vi "Open Sensors and Actuators.vi"   [LabVIEW 2014]
uses:
  <vilib>/Rock Robotics/SystemInterfaces/DIO/FPGA_DIOPWMChannel.ctl
  <vilib>/Rock Robotics/SystemInterfaces/AI/FPGA_AIChannel.ctl
  <vilib>/Rock Robotics/WPI/Joystick/WPI_JoystickDeviceEnum.ctl
  <vilib>/Rock Robotics/SystemInterfaces/DIO/FPGA_DIOChannel.ctl
  <vilib>/Rock Robotics/WPI/Solenoid/WPI_SolenoidChannel.ctl
  <vilib>/Rock Robotics/SystemInterfaces/Typedef/FPGA_TypedefAnalogModule.ctl
  <vilib>/Rock Robotics/WPI/MotorControl/WPI_MotorControlOpen Talon.vi
  <vilib>/Rock Robotics/WPI/Counter/WPI_CounterDigitalInputToDigitalSource.vi
  <vilib>/Rock Robotics/WPI/Solenoid/WPI_SolenoidOpenSingle.vi
  <vilib>/Rock Robotics/WPI/Counter/WPI_CounterOpen UpDown Mode.vi
  <vilib>/Rock Robotics/WPI/Switch/WPI_SwitchOpenLimit.vi
  Global RefNums.vi
  <vilib>/Rock Robotics/WPI/Compressor/WPI_CompressorGetSetRefNum.vi
  _Dependencies/NavX/navX-MXP IMU.lvlib
types:
  T1 = typedef "FPGA_AIChannel.ctl" = enum8{"AI 0", "AI 1", "AI 2", "AI 3", "AI MXP 0", "AI MXP 1", "AI MXP 2", "AI MXP 3", "Invalid"}
  T2 = typedef "FPGA_TypedefAnalogModule.ctl" = enum16{"Controller 1"}
  T3 = typedef "FPGA_DIOPWMChannel.ctl" = enum8{"PWM 0", "PWM 1", "PWM 2", "PWM 3", "PWM 4", "PWM 5", "PWM 6", "PWM 7", "PWM 8", "PWM 9", "PWM MXP 0", "PWM MXP 1", "PWM MXP 2", "PWM MXP 3", "PWM MXP 4", "PWM MXP 5", "PWM MXP 6", "PWM MXP 7", "PWM MXP 8", "PWM MXP 9", "Invalid"}
  T4 = typedef "FPGA_DIOChannel.ctl" = enum8{"DIO 0", "DIO 1", "DIO 2", "DIO 3", "DIO 4", "DIO 5", "DIO 6", "DIO 7", "DIO 8", "DIO 9", "DIO MXP 0", "DIO MXP 1", "DIO MXP 2", "DIO MXP 3", "DIO MXP 4", "DIO MXP 5", "DIO MXP 6", "DIO MXP 7", "DIO MXP 8", "DIO MXP 9", "DIO MXP 10", "DIO MXP 11", "DIO MXP 12", "DIO MXP 13", "DIO MXP 14", "DIO MXP 15", "Invalid"}
  T5 = enum16{"Rising Edge", "Falling Edge", "Raising & Falling Edge", "Disabled"}
  T6 = typedef "WPI_SolenoidChannel.ctl" = enum8{"Solenoid 0", "Solenoid 1", "Solenoid 2", "Solenoid 3", "Solenoid 4", "Solenoid 5", "Solenoid 6", "Solenoid 7", "Invalid"}
  T7 = typedef "WPI_JoystickDeviceEnum.ctl" = enum16{"USB 0", "USB 1", "USB 2", "USB 3", "USB 4", "USB 5"}
  T8 = typedef "WPI_MotorControlDeviceRef.ctl" = cluster{"DeviceStatus":errorcluster, "Type":T9, "PWM":cluster{"Controller":T10, "PWM Channel":T3, "DeadBand":T11}, "CAN":cluster{"Device Number":u8, "Control Mode":T12, "Semaphore":T13, "Max Vout":dbl, "TalonSRX Control Mode":T14}, "Invert":bool, "TransformRef":T15, "InvTransformRef":T15}
  T9 = typedef "WPI_MotorControlType.ctl" = enum16{"PWM", "CAN", "CANTalonSRX"}
  T10 = typedef "FPGA_TypedefDigitalModule.ctl" = enum16{"Controller 1"}
  T11 = typedef "WPI_PWMDeadband.ctl" = cluster{"Name":string, "maxPositivePwm":i32, "minPositivePwm":i32, "centerPwm":i32, "maxNegativePwm":i32, "minNegativePwm":i32, "angularRange":u16}
  T12 = typedef "WPI_CANJaguar_ControlMode.ctl" = enum8{"Percent VBus", "Current", "Speed", "Position", "Voltage"}
  T13 = typedef "Semaphore RefNum" = refnum<k1>
  T14 = typedef "WPI_CANTalonSRX_APIControlMode.ctl" = enum8{"Percent VBus", "Speed", "Position", "Slave", "Unchanged / Invalid"}
  T15 = typedef "WPI_PWMTransform_ConPane.ctl" = refnum<vi>
  T16 = typedef "WPI_DigitalInputDevRef.ctl" = cluster{"DevStatus":errorcluster, "DIO Channel":T4, "Controller":T10}
  T17 = typedef "FPGA_CounterEncoderSourceConvertionLVSourceType.ctl" = cluster{"DevStatus":errorcluster, "AnalogTriggerMode?":bool, "DigitalMode":cluster{"Controller":T10, "DIO Channel":T18}, "AnalogTriggerMode":cluster{"AnalogTriggerIndex":T19, "OutputType":T20}}
  T18 = typedef "FPGA_DIODigitalSourceChannel.ctl" = enum8{"DIO 0", "DIO 1", "DIO 2", "DIO 3", "DIO 4", "DIO 5", "DIO 6", "DIO 7", "DIO 8", "DIO 9", "DIO MXP 0", "DIO MXP 1", "DIO MXP 2", "DIO MXP 3", "DIO MXP 4", "DIO MXP 5", "DIO MXP 6", "DIO MXP 7", "DIO MXP 8", "DIO MXP 9", "DIO MXP 10", "DIO MXP 11", "DIO MXP 12", "DIO MXP 13", "DIO MXP 14", "DIO MXP 15", "Disabled"}
  T19 = typedef "FPGA_AnalogTriggerIndex.ctl" = enum8{"Trig 0", "Trig 1", "Trig 2", "Trig 3", "Trig 4", "Trig 5", "Trig 6", "Trig 7", "Invalid"}
  T20 = typedef "FPGA_AnalogTriggerOutType.ctl" = enum16{"InWindow", "TriggerState", "Rising", "Falling"}
  T21 = typedef "WPI_EncoderDevRef.ctl" = cluster{"DevStatus":errorcluster, "EncoderIndex":T22, "CounterIndex":T23, "DistancePerCount":dbl, "Decoding Type":T24}
  T22 = typedef "FPGA_EncoderIdx.ctl" = enum8{"Enc 0", "Enc 1", "Enc 2", "Enc 3", "Enc 4", "Enc 5", "Enc 6", "Enc 7", "Invalid"}
  T23 = typedef "FPGA_CounterCtrSystemIndex.ctl" = enum8{"Ctr 0", "Ctr 1", "Ctr 2", "Ctr 3", "Ctr 4", "Ctr 5", "Ctr 6", "Ctr 7", "Invalid"}
  T24 = typedef "WPI_EncoderType.ctl" = enum16{"1x", "2x", "4x"}
  T25 = typedef "navX-MXP IMU.lvlib/navX Device TypeDef.ctl" = cluster{"navX Interface Protocol":T26, "navX Interface Protocol TypeDefs":cluster{"SPIDevRef":T27, "I2CDevRef":T29}, "navX System Information":cluster{"Board Information":T31, "Status":T32, "Offsets":T36}, "navX Common Information":cluster{"Update Rate (4Hz-60Hz)":T37, "refnum name":string, "error":errorcluster}}
  T26 = typedef "navX-MXP IMU.lvlib/navX Interface Protocol.ctl" = enum16{"SPI", "I2C"}
  T27 = typedef "WPI_SPIDevRef.ctl" = cluster{"DevStatus":errorcluster, "Handle":i32, "Controller":T10, "SPI Bus":T28}
  T28 = typedef "spi_bus.ctl" = enum16{"SPI On-Board, CS0", "SPI On-Board, CS1", "SPI On-Board, CS2", "SPI On-Board, CS3", "SPI MXP", "Invalid"}
  T29 = typedef "WPI_I2CDevRef.ctl" = cluster{"DevStatus":errorcluster, "Controller":T10, "Device Address":u8, "Handle":i32, "I2C Bus":T30}
  T30 = typedef "i2c_bus.ctl" = enum16{"I2C On-Board", "I2C MXP", "Invalid"}
  T31 = typedef "navX-MXP IMU.lvlib/navX Board Information.ctl" = cluster{"WhoAmI (50 | 0x32)":u8, "Board Revision":u8, "Firmware Major Version":u8, "Firmware Minor Version":u8}
  T32 = typedef "navX-MXP IMU.lvlib/navX Status Data.ctl" = cluster{"Update Rate Hz":u8, "Accelerometer Full-Scale Range":u8, "Gyro Full-Scale Range":u16, "NAVX_OP_STATUS":T33, "NAVX_CAL_STATUS":T34, "NAVX_SELFTEST_STATUS":u8, "NAVX_SENSOR_STATUS":T35}
  T33 = typedef "navX-MXP IMU.lvlib/navX NAVX_OP_STATUS.ctl" = u8
  T34 = typedef "navX-MXP IMU.lvlib/navX NAVX_CAL_STATUS.ctl" = u8
  T35 = typedef "navX-MXP IMU.lvlib/navX NAVX_SENSOR_STATUS.ctl" = cluster{"MOVING":bool, "YAW_STABLE":bool, "MAG_DISTURBANCE":bool, "ALTITUDE_VALID":bool, "SEALEVEL_PRESS_SET":bool, "FUSED_HEADING_VALID":bool}
  T36 = typedef "navX-MXP IMU.lvlib/navX Offsets Data.ctl" = cluster{"Yaw":dbl, "Quat W":dbl, "Quat X":dbl, "Quat Y":dbl, "Quat Z":dbl}
  T37 = typedef "navX-MXP IMU.lvlib/navX Update Rate.ctl" = u8
  T38 = typedef "WPI_JoystickDevRef.ctl" = cluster{"Device":T7}
  T39 = typedef "WPI_AnalogChannelDevRef.ctl" = cluster{"DevStatus":errorcluster, "Controller":T2, "Analog Channel":T1}
  T40 = typedef "WPI_SolenoidDevRef.ctl" = cluster{"DevStatus":errorcluster, "Pneumatics Control Module":u8, "Forward Solenoid Channel":T6, "Reverse Solenoid Channel":T6}
  T41 = typedef "WPI_CounterDevRef.ctl" = cluster{"DevStatus":errorcluster, "CntIndex":T23}
  T42 = typedef "WPI_CompressorDevRef.ctl" = cluster{"DevStatus":errorcluster, "Pneumatics Control Module":u8}
  T43 = typedef "WPI_SwitchDevRef.ctl" = cluster{"DevStatus":errorcluster, "DIO Channel":T4, "Controller":T10, "CntIndex":T23, "Normally Closed":bool}
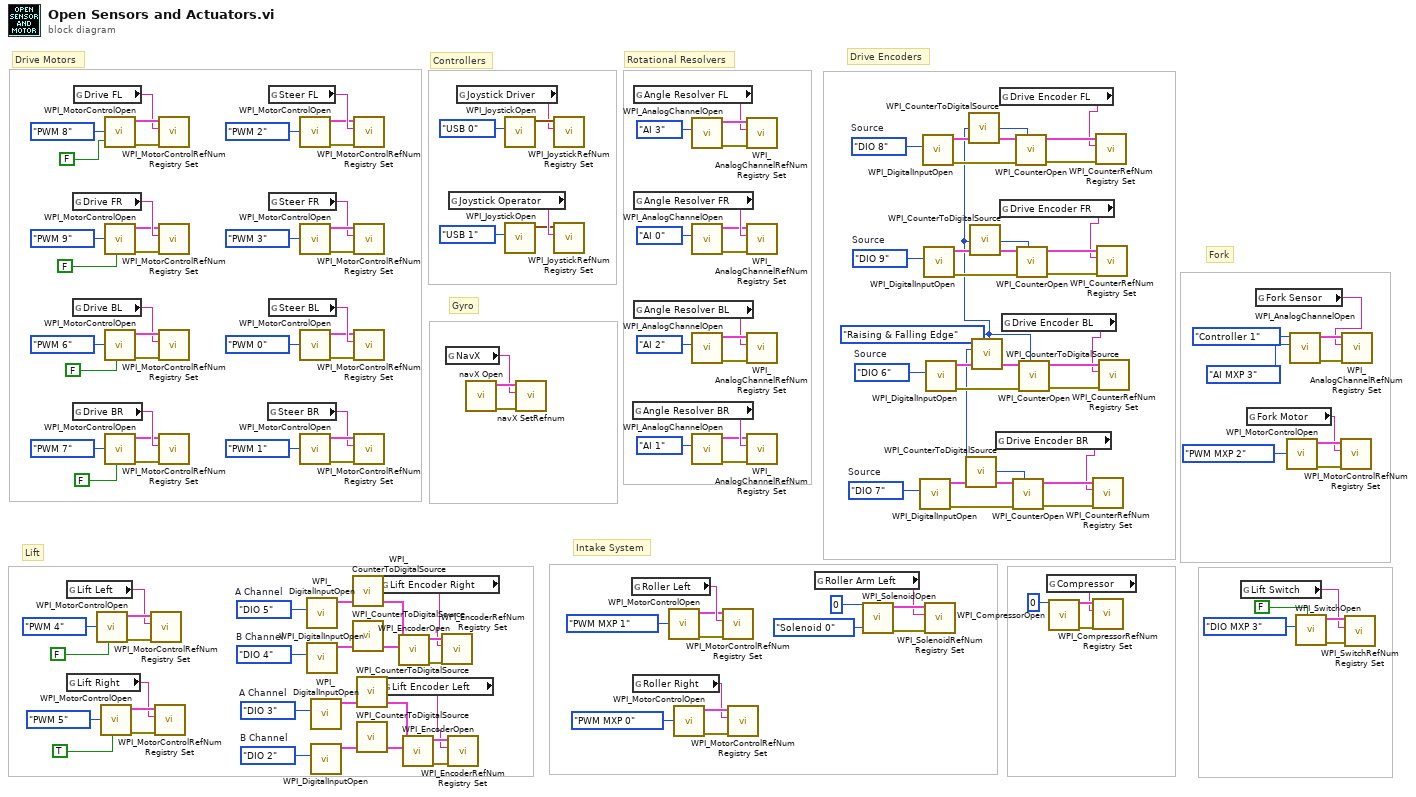
[diagram p0: block diagram]
diagram:
  w15 = T5."Raising & Falling Edge" ("UpEdge")
  w25 = FPGA_DIOChannel."DIO 7"  # Source
  w32 = FPGA_DIOChannel."DIO 6"  # Source
  w39 = FPGA_DIOChannel."DIO 9"  # Source
  w67 = FPGA_DIOChannel."DIO 2"  # B Channel
  w66 = FPGA_DIOChannel."DIO 3"  # A Channel
  w73 = FPGA_DIOChannel."DIO 4"  # B Channel
  w72 = FPGA_DIOChannel."DIO 5"  # A Channel
  w94 = FPGA_DIOChannel."DIO 8"  # Source
  # "Fork"
  # "Intake System"
  # "Gyro"
  # "Drive Encoders"
  # "Lift"
  # "Drive Motors"
  # "Controllers"
  # "Rotational Resolvers"
  n1 = global read "Global RefNums.vi" "Lift Left"() -> (w83:string)
  n2 = global read "Global RefNums.vi" "Lift Right"() -> (w79:string)
  n3 = global read "Global RefNums.vi" "Drive FR"() -> (w141:string)
  n4 = global read "Global RefNums.vi" "Drive BL"() -> (w136:string)
  n5 = global read "Global RefNums.vi" "Drive BR"() -> (w133:string)
  n6 = global read "Global RefNums.vi" "Drive FL"() -> (w144:string)
  n7 = call-poly <vilib>:"WPI_MotorControlOpen.vi"("Invert"=FALSE, "PWM Channel"=FPGA_DIOPWMChannel."PWM 4") -> ("error out"=w84:errorcluster, "MotorControlDeviceRef"=w85:T8)  [unwired: 8 in]
  n8 = call-poly <vilib>:"WPI_MotorControlOpen.vi"("Invert"=TRUE, "PWM Channel"=FPGA_DIOPWMChannel."PWM 5") -> ("error out"=w80:errorcluster, "MotorControlDeviceRef"=w81:T8)  [unwired: 8 in]
  n9 = call-poly <vilib>:"WPI_MotorControlOpen.vi"("Invert"=FALSE, "PWM Channel"=FPGA_DIOPWMChannel."PWM 8") -> ("error out"=w145:errorcluster, "MotorControlDeviceRef"=w146:T8)  [unwired: 8 in]
  n10 = call-poly <vilib>:"WPI_MotorControlOpen.vi"("Invert"=FALSE, "PWM Channel"=FPGA_DIOPWMChannel."PWM 9") -> ("error out"=w140:errorcluster, "MotorControlDeviceRef"=w139:T8)  [unwired: 8 in]
  n11 = call-poly <vilib>:"WPI_MotorControlOpen.vi"("Invert"=FALSE, "PWM Channel"=FPGA_DIOPWMChannel."PWM 6") -> ("error out"=w137:errorcluster, "MotorControlDeviceRef"=w138:T8)  [unwired: 8 in]
  n12 = call-poly <vilib>:"WPI_MotorControlOpen.vi"("Invert"=FALSE, "PWM Channel"=FPGA_DIOPWMChannel."PWM 7") -> ("error out"=w132:errorcluster, "MotorControlDeviceRef"=w131:T8)  [unwired: 8 in]
  n13 = call <vilib>:"WPI_MotorControlRefNum Registry Set.vi"("error in (no error)"=w84, "refnum name"=w83, "MotorControlDevRef"=w85) -> ()  [unwired: 7 in, 2 out]
  n14 = call <vilib>:"WPI_MotorControlRefNum Registry Set.vi"("error in (no error)"=w80, "refnum name"=w79, "MotorControlDevRef"=w81) -> ()  [unwired: 7 in, 2 out]
  n15 = call <vilib>:"WPI_MotorControlRefNum Registry Set.vi"("error in (no error)"=w145, "refnum name"=w144, "MotorControlDevRef"=w146) -> ()  [unwired: 7 in, 2 out]
  n16 = call <vilib>:"WPI_MotorControlRefNum Registry Set.vi"("error in (no error)"=w140, "refnum name"=w141, "MotorControlDevRef"=w139) -> ()  [unwired: 7 in, 2 out]
  n17 = call <vilib>:"WPI_MotorControlRefNum Registry Set.vi"("error in (no error)"=w137, "refnum name"=w136, "MotorControlDevRef"=w138) -> ()  [unwired: 7 in, 2 out]
  n18 = call <vilib>:"WPI_MotorControlRefNum Registry Set.vi"("error in (no error)"=w132, "refnum name"=w133, "MotorControlDevRef"=w131) -> ()  [unwired: 7 in, 2 out]
  n19 = global read "Global RefNums.vi" "Steer BR"() -> (w128:string)
  n20 = global read "Global RefNums.vi" "Steer FL"() -> (w117:string)
  n21 = global read "Global RefNums.vi" "Steer FR"() -> (w120:string)
  n22 = global read "Global RefNums.vi" "Steer BL"() -> (w125:string)
  n23 = call-poly <vilib>:"WPI_MotorControlOpen.vi"("PWM Channel"=FPGA_DIOPWMChannel."PWM 2") -> ("error out"=w116:errorcluster, "MotorControlDeviceRef"=w115:T8)  [unwired: 9 in]
  n24 = call-poly <vilib>:"WPI_MotorControlOpen.vi"("PWM Channel"=FPGA_DIOPWMChannel."PWM 3") -> ("error out"=w121:errorcluster, "MotorControlDeviceRef"=w122:T8)  [unwired: 9 in]
  n25 = call-poly <vilib>:"WPI_MotorControlOpen.vi"("PWM Channel"=FPGA_DIOPWMChannel."PWM 0") -> ("error out"=w124:errorcluster, "MotorControlDeviceRef"=w123:T8)  [unwired: 9 in]
  n26 = call-poly <vilib>:"WPI_MotorControlOpen.vi"("PWM Channel"=FPGA_DIOPWMChannel."PWM 1") -> ("error out"=w129:errorcluster, "MotorControlDeviceRef"=w130:T8)  [unwired: 9 in]
  n27 = call <vilib>:"WPI_DigitalInputOpen.vi"("DIO Channel"=w72) -> ("DigitalInputDevRef"=w69:T16)  [unwired: 2 in, 8 out]
  n28 = call <vilib>:"WPI_DigitalInputOpen.vi"("DIO Channel"=w73) -> ("DigitalInputDevRef"=w70:T16)  [unwired: 2 in, 8 out]
  n29 = call <vilib>:"WPI_DigitalInputOpen.vi"("DIO Channel"=w66) -> ("DigitalInputDevRef"=w63:T16)  [unwired: 2 in, 8 out]
  n30 = call <vilib>:"WPI_DigitalInputOpen.vi"("DIO Channel"=w67) -> ("DigitalInputDevRef"=w64:T16)  [unwired: 2 in, 8 out]
  n31 = call-poly <vilib>:"WPI_CounterToDigitalSource.vi"("DigitalInputDevRef"=w69) -> ("Digital Source"=w68:T17)  [unwired: 6 out]
  n32 = call-poly <vilib>:"WPI_CounterToDigitalSource.vi"("DigitalInputDevRef"=w70) -> ("Digital Source"=w71:T17)  [unwired: 6 out]
  n33 = call <vilib>:"WPI_MotorControlRefNum Registry Set.vi"("error in (no error)"=w116, "refnum name"=w117, "MotorControlDevRef"=w115) -> ()  [unwired: 7 in, 2 out]
  n34 = call <vilib>:"WPI_MotorControlRefNum Registry Set.vi"("error in (no error)"=w121, "refnum name"=w120, "MotorControlDevRef"=w122) -> ()  [unwired: 7 in, 2 out]
  n35 = call <vilib>:"WPI_MotorControlRefNum Registry Set.vi"("error in (no error)"=w124, "refnum name"=w125, "MotorControlDevRef"=w123) -> ()  [unwired: 7 in, 2 out]
  n36 = call <vilib>:"WPI_MotorControlRefNum Registry Set.vi"("error in (no error)"=w129, "refnum name"=w128, "MotorControlDevRef"=w130) -> ()  [unwired: 7 in, 2 out]
  n37 = call-poly <vilib>:"WPI_CounterToDigitalSource.vi"("DigitalInputDevRef"=w63) -> ("Digital Source"=w62:T17)  [unwired: 6 out]
  n38 = call-poly <vilib>:"WPI_CounterToDigitalSource.vi"("DigitalInputDevRef"=w64) -> ("Digital Source"=w65:T17)  [unwired: 6 out]
  n39 = global read "Global RefNums.vi" "Lift Encoder Right"() -> (w56:string)
  n40 = global read "Global RefNums.vi" "Lift Encoder Left"() -> (w57:string)
  n41 = call <vilib>:"WPI_EncoderOpen.vi"("BSource"=w71, "ASource"=w68) -> ("error out"=w61:errorcluster, "EncoderDevRef"=w60:T21)  [unwired: 6 in, 2 out]
  n42 = call <vilib>:"WPI_EncoderOpen.vi"("BSource"=w65, "ASource"=w62) -> ("error out"=w59:errorcluster, "EncoderDevRef"=w58:T21)  [unwired: 6 in, 2 out]
  n43 = call <vilib>:"WPI_EncoderRefNum Registry Set.vi"("error in (no error)"=w61, "refnum name"=w56, "EncoderDevRef"=w60) -> ()  [unwired: 7 in, 2 out]
  n44 = global read "Global RefNums.vi" "NavX"() -> (w86:string)
  n45 = call <vilib>:"WPI_EncoderRefNum Registry Set.vi"("error in (no error)"=w59, "refnum name"=w57, "EncoderDevRef"=w58) -> ()  [unwired: 7 in, 2 out]
  n46 = global read "Global RefNums.vi" "Joystick Operator"() -> (w113:string)
  n47 = global read "Global RefNums.vi" "Joystick Driver"() -> (w114:string)
  n48 = call "navX Open.vi"() -> ("error out"=w88:errorcluster, "navX Device TypeDef"=w87:T25)  [unwired: 9 in, 1 out]
  n49 = call <vilib>:"WPI_JoystickOpen.vi"("JoystickDevice"=WPI_JoystickDeviceEnum."USB 0") -> ("JoystickDevRef"=w147:T38)  [unwired: 10 in]
  n50 = call <vilib>:"WPI_JoystickOpen.vi"("JoystickDevice"=WPI_JoystickDeviceEnum."USB 1") -> ("JoystickDevRef"=w112:T38)  [unwired: 10 in]
  n51 = call "navX SetRefnum.vi"("error in (no error)"=w88, "refnum name"=w86, "navX Device TypeDef"=w87) -> ()  [unwired: 7 in, 2 out]
  n52 = call <vilib>:"WPI_JoystickRefNum Registry Set.vi"("refnum name"=w114, "JoystickDevRef"=w147) -> ()  [unwired: 8 in, 2 out]
  n53 = call <vilib>:"WPI_JoystickRefNum Registry Set.vi"("refnum name"=w113, "JoystickDevRef"=w112) -> ()  [unwired: 8 in, 2 out]
  n54 = global read "Global RefNums.vi" "Roller Left"() -> (w52:string)
  n55 = global read "Global RefNums.vi" "Angle Resolver BR"() -> (w100:string)
  n56 = global read "Global RefNums.vi" "Roller Right"() -> (w47:string)
  n57 = global read "Global RefNums.vi" "Angle Resolver FL"() -> (w111:string)
  n58 = global read "Global RefNums.vi" "Angle Resolver FR"() -> (w108:string)
  n59 = global read "Global RefNums.vi" "Angle Resolver BL"() -> (w103:string)
  n60 = call-poly <vilib>:"WPI_MotorControlOpen.vi"("PWM Channel"=FPGA_DIOPWMChannel."PWM MXP 1") -> ("error out"=w51:errorcluster, "MotorControlDeviceRef"=w50:T8)  [unwired: 9 in]
  n61 = call-poly <vilib>:"WPI_MotorControlOpen.vi"("PWM Channel"=FPGA_DIOPWMChannel."PWM MXP 0") -> ("error out"=w48:errorcluster, "MotorControlDeviceRef"=w49:T8)  [unwired: 9 in]
  n62 = call <vilib>:"WPI_AnalogChannelOpen.vi"("Analog Channel"=FPGA_AIChannel."AI 3") -> ("error out"=w149:errorcluster, "AIDeviceRef"=w148:T39)  [unwired: 9 in]
  n63 = call <vilib>:"WPI_AnalogChannelOpen.vi"("Analog Channel"=FPGA_AIChannel."AI 0") -> ("error out"=w106:errorcluster, "AIDeviceRef"=w107:T39)  [unwired: 9 in]
  n64 = call <vilib>:"WPI_AnalogChannelOpen.vi"("Analog Channel"=FPGA_AIChannel."AI 2") -> ("error out"=w105:errorcluster, "AIDeviceRef"=w104:T39)  [unwired: 9 in]
  n65 = call <vilib>:"WPI_AnalogChannelOpen.vi"("Analog Channel"=FPGA_AIChannel."AI 1") -> ("error out"=w98:errorcluster, "AIDeviceRef"=w99:T39)  [unwired: 9 in]
  n66 = call <vilib>:"WPI_MotorControlRefNum Registry Set.vi"("error in (no error)"=w51, "refnum name"=w52, "MotorControlDevRef"=w50) -> ()  [unwired: 7 in, 2 out]
  n67 = call <vilib>:"WPI_MotorControlRefNum Registry Set.vi"("error in (no error)"=w48, "refnum name"=w47, "MotorControlDevRef"=w49) -> ()  [unwired: 7 in, 2 out]
  n68 = call <vilib>:"WPI_AnalogChannelRefNum Registry Set.vi"("error in (no error)"=w149, "refnum name"=w111, "AIDeviceRef"=w148) -> ()  [unwired: 7 in, 2 out]
  n69 = call <vilib>:"WPI_AnalogChannelRefNum Registry Set.vi"("error in (no error)"=w106, "refnum name"=w108, "AIDeviceRef"=w107) -> ()  [unwired: 7 in, 2 out]
  n70 = call <vilib>:"WPI_AnalogChannelRefNum Registry Set.vi"("error in (no error)"=w105, "refnum name"=w103, "AIDeviceRef"=w104) -> ()  [unwired: 7 in, 2 out]
  n71 = call <vilib>:"WPI_AnalogChannelRefNum Registry Set.vi"("error in (no error)"=w98, "refnum name"=w100, "AIDeviceRef"=w99) -> ()  [unwired: 7 in, 2 out]
  n72 = global read "Global RefNums.vi" "Roller Arm Left"() -> (w41:string)
  n73 = call-poly <vilib>:"WPI_SolenoidOpen.vi"("Solenoid Channel"=WPI_SolenoidChannel."Solenoid 0", "Pneumatics Control Module (0)"=u8 0) -> ("error out"=w44:errorcluster, "SolenoidDevRef"=w45:T40)  [unwired: 8 in]
  n74 = call <vilib>:"WPI_DigitalInputOpen.vi"("DIO Channel"=w25) -> ("error out"=w21:errorcluster, "DigitalInputDevRef"=w24:T16)  [unwired: 2 in, 7 out]
  n75 = call <vilib>:"WPI_DigitalInputOpen.vi"("DIO Channel"=w94) -> ("error out"=w90:errorcluster, "DigitalInputDevRef"=w93:T16)  [unwired: 2 in, 7 out]
  n76 = call <vilib>:"WPI_DigitalInputOpen.vi"("DIO Channel"=w39) -> ("error out"=w35:errorcluster, "DigitalInputDevRef"=w38:T16)  [unwired: 2 in, 7 out]
  n77 = call <vilib>:"WPI_SolenoidRefNum Registry Set.vi"("error in (no error)"=w44, "refnum name"=w41, "SolenoidDevRef"=w45) -> ()  [unwired: 7 in, 2 out]
  n78 = call <vilib>:"WPI_DigitalInputOpen.vi"("DIO Channel"=w32) -> ("error out"=w28:errorcluster, "DigitalInputDevRef"=w31:T16)  [unwired: 2 in, 7 out]
  n79 = call-poly <vilib>:"WPI_CounterToDigitalSource.vi"("DigitalInputDevRef"=w24) -> ("Digital Source"=w26:T17)  [unwired: 6 out]
  n80 = call-poly <vilib>:"WPI_CounterToDigitalSource.vi"("DigitalInputDevRef"=w93) -> ("Digital Source"=w95:T17)  [unwired: 6 out]
  n81 = call-poly <vilib>:"WPI_CounterToDigitalSource.vi"("DigitalInputDevRef"=w38) -> ("Digital Source"=w40:T17)  [unwired: 6 out]
  n82 = call-poly <vilib>:"WPI_CounterToDigitalSource.vi"("DigitalInputDevRef"=w31) -> ("Digital Source"=w33:T17)  [unwired: 6 out]
  n83 = global read "Global RefNums.vi" "Drive Encoder BR"() -> (w20:string)
  n84 = global read "Global RefNums.vi" "Drive Encoder FL"() -> (w89:string)
  n85 = global read "Global RefNums.vi" "Drive Encoder FR"() -> (w34:string)
  n86 = global read "Global RefNums.vi" "Drive Encoder BL"() -> (w27:string)
  n87 = call-poly <vilib>:"WPI_CounterOpen.vi"("UpEdge"=w15, "error in (no error)"=w21, "Up Source"=w26) -> ("error out"=w22:errorcluster, "CounterDevRef"=w23:T41)  [unwired: 4 in, 3 out]
  n88 = call-poly <vilib>:"WPI_CounterOpen.vi"("UpEdge"=w15, "error in (no error)"=w90, "Up Source"=w95) -> ("error out"=w91:errorcluster, "CounterDevRef"=w92:T41)  [unwired: 4 in, 3 out]
  n89 = call-poly <vilib>:"WPI_CounterOpen.vi"("UpEdge"=w15, "error in (no error)"=w35, "Up Source"=w40) -> ("error out"=w36:errorcluster, "CounterDevRef"=w37:T41)  [unwired: 4 in, 3 out]
  n90 = call-poly <vilib>:"WPI_CounterOpen.vi"("UpEdge"=w15, "error in (no error)"=w28, "Up Source"=w33) -> ("error out"=w29:errorcluster, "CounterDevRef"=w30:T41)  [unwired: 4 in, 3 out]
  n91 = global read "Global RefNums.vi" "Compressor"() -> (w16:string)
  n92 = call <vilib>:"WPI_CompressorOpen.vi"("Pneumatics Control Module (0)"=u8 0) -> ("CompressorDevRef"=w19:T42, "error out"=w18:errorcluster)  [unwired: 13 in]
  n93 = call <vilib>:"WPI_CounterRefNum Registry Set.vi"("error in (no error)"=w22, "refnum name"=w20, "CounterDevRef"=w23) -> ()  [unwired: 7 in, 2 out]
  n94 = call <vilib>:"WPI_CompressorRefNum Registry Set.vi"("error in (no error)"=w18, "refnum name"=w16, "CompressorDevRef"=w19) -> ()  [unwired: 7 in, 2 out]
  n95 = call <vilib>:"WPI_CounterRefNum Registry Set.vi"("error in (no error)"=w91, "refnum name"=w89, "CounterDevRef"=w92) -> ()  [unwired: 7 in, 2 out]
  n96 = call <vilib>:"WPI_CounterRefNum Registry Set.vi"("error in (no error)"=w36, "refnum name"=w34, "CounterDevRef"=w37) -> ()  [unwired: 7 in, 2 out]
  n97 = call <vilib>:"WPI_CounterRefNum Registry Set.vi"("error in (no error)"=w29, "refnum name"=w27, "CounterDevRef"=w30) -> ()  [unwired: 7 in, 2 out]
  n98 = global read "Global RefNums.vi" "Lift Switch"() -> (w11:string)
  n99 = global read "Global RefNums.vi" "Fork Motor"() -> (w7:string)
  n100 = global read "Global RefNums.vi" "Fork Sensor"() -> (w1:string)
  n101 = call-poly <vilib>:"WPI_MotorControlOpen.vi"("PWM Channel"=FPGA_DIOPWMChannel."PWM MXP 2") -> ("error out"=w8:errorcluster, "MotorControlDeviceRef"=w9:T8)  [unwired: 9 in]
  n102 = call <vilib>:"WPI_AnalogChannelOpen.vi"("Analog Channel"=FPGA_AIChannel."AI MXP 3", "Controller"=FPGA_TypedefAnalogModule."Controller 1") -> ("error out"=w4:errorcluster, "AIDeviceRef"=w5:T39)  [unwired: 8 in]
  n103 = call-poly <vilib>:"WPI_SwitchOpen.vi"("Normally Closed"=FALSE, "DIO Channel"=FPGA_DIOChannel."DIO MXP 3") -> ("error out"=w14:errorcluster, "SwitchDevRef"=w13:T43)  [unwired: 8 in]
  n104 = call <vilib>:"WPI_MotorControlRefNum Registry Set.vi"("error in (no error)"=w8, "refnum name"=w7, "MotorControlDevRef"=w9) -> ()  [unwired: 7 in, 2 out]
  n105 = call <vilib>:"WPI_AnalogChannelRefNum Registry Set.vi"("error in (no error)"=w4, "refnum name"=w1, "AIDeviceRef"=w5) -> ()  [unwired: 7 in, 2 out]
  n106 = call <vilib>:"WPI_SwitchRefNum Registry Set.vi"("error in (no error)"=w14, "refnum name"=w11, "SwitchDevRef"=w13) -> ()  [unwired: 7 in, 2 out]
